vi "ZENTYPE.vi"() -> ()   [LabVIEW 2020]
panel:
  in  "ZENTYPE":string
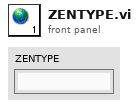
[diagram p1: front panel]
diagram:
